vi "RadiusNeighborsRegressor.vi"(8 "error in":errorcluster) -> (0 "error out":errorcluster, 3 "out":refnum<class "RadiusNeighborsRegressor.lvclass">)   [LabVIEW 2020]
doc: "Regression based on neighbors within a fixed radius.\n\n The target is predicted by local interpolation of the targets\n associated of the nearest neighbors in the training set.\n\n Read more in the :ref:`User Guide <regression>`.\n\n .. versionadded:: 0.9\n\n Parameters\n ----------\n radius : float, default=1.0\n Range of parameter space to use by default for :meth:`radius_neighbors`\n queries.\n\n weights : {'uniform', 'distance'} or callable, default='uniform'\n weight function used in prediction. Possible values:\n\n - 'uniform' : uniform weights. All points in each neighborhood\n are weighted equally.\n - 'distance' : weight points by the inverse of their distance.\n in this case, closer neighbors of a query point will have a\n greater influence than neighbors which are further away.\n - [callable] : a user-defined function which accepts an\n array of distances, and returns an array of the same shape\n containing the weights.\n\n Uniform weights are used by default.\n\n algorithm : {'auto', 'ball_tree', 'kd_tree', 'brute'}, default='auto'\n Algorithm used to compute the nearest neighbors:\n\n - 'ball_tree' will use :class:`BallTree`\n - 'kd_tree' will use :class:`KDTree`\n - 'brute' will use a brute-force search.\n - 'auto' will attempt to decide the most appropriate algorithm\n based on the values passed to :meth:`fit` method.\n\n Note: fitting on sparse input will override the setting of\n this parameter, using brute force.\n\n leaf_size : int, default=30\n Leaf size passed to BallTree or KDTree. This can affect the\n speed of the construction and query, as well as the memory\n required to store the tree. The optimal value depends on the\n nature of the problem.\n\n p : int, default=2\n Power parameter for the Minkowski metric. When p = 1, this is\n equivalent to using manhattan_distance (l1), and euclidean_distance\n (l2) for p = 2. For arbitrary p, minkowski_distance (l_p) is used.\n\n metric : str or callable, default='minkowski'\n the distance metric to use for the tree. The default metric is\n minkowski, and with p=2 is equivalent to the standard Euclidean\n metric. See the documentation of :class:`DistanceMetric` for a\n list of available metrics.\n If metric is \"precomputed\", X is assumed to be a distance matrix and\n must be square during fit. X may be a :term:`sparse graph`,\n in which case only \"nonzero\" elements may be considered neighbors.\n\n metric_params : dict, default=None\n Additional keyword arguments for the metric function.\n\n n_jobs : int, default=None\n The number of parallel jobs to run for neighbors search.\n ``None`` means 1 unless in a :obj:`joblib.parallel_backend` context.\n ``-1`` means using all processors. See :term:`Glossary <n_jobs>`\n for more details.\n\n Attributes\n ----------\n effective_metric_ : str or callable\n The distance metric to use. It will be same as the `metric` parameter\n or a synonym of it, e.g. 'euclidean' if the `metric` parameter set to\n 'minkowski' and `p` parameter set to 2.\n\n effective_metric_params_ : dict\n Additional keyword arguments for the metric function. For most metrics\n will be same with `metric_params` parameter, but may also contain the\n `p` parameter value if the `effective_metric_` attribute is set to\n 'minkowski'.\n\n n_samples_fit_ : int\n Number of samples in the fitted data.\n\n \nAvailable methods:\nRadius Neighbors\nRadius Neighbors Graph\nFit\nPredict\nScore\nGet Attributes\nGet Params\nSet Params"
uses:
  RadiusNeighborsRegressor.lvclass
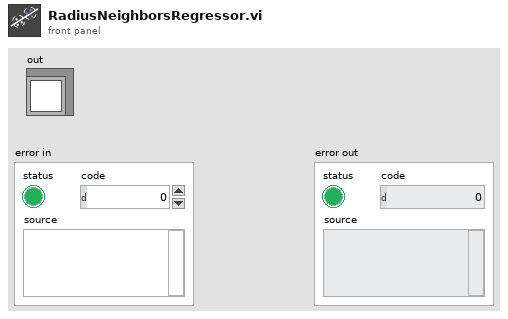
[diagram p1: front panel]
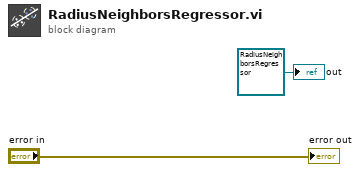
[diagram p0: block diagram]
diagram:
  "out" <- refnum<class "RadiusNeighborsRegressor.lvclass"> refnum ("model")
  "error out" <- "error in"
